vi "RSA FIX.vi"() -> ()   [LabVIEW 2017]
uses:
  <vilib>/Enthought/Python Integration Toolkit/api/Unpack String.vi
  <vilib>/Enthought/Python Integration Toolkit/Python Integration Toolkit.lvlib
panel:
  out "chiptertext":string
  out "plaintext":string
  in  "chipertext":string
  out "Array 2":string[](array[string])
  in  "plaintext":string
  out "error out 3":errorcluster
  out "Array":string[](array[string])
  out "?":string="DESKRIPSI"
  out "error out 2":errorcluster
  out "?":string="DESKRIPSI"
  out "Totient":i64
  in  "e":i64
  out "N":i64
  in  "q":i64
  in  "p":i64
  out "d":i64
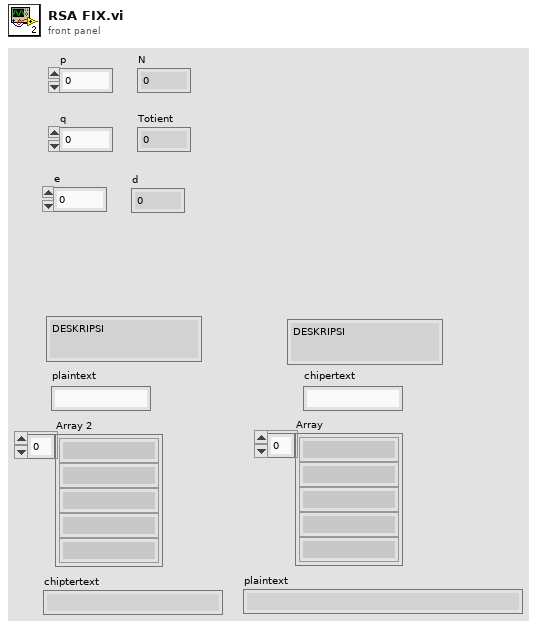
[diagram p1: front panel]
types:
  T1 = typedef "Python Integration Toolkit.lvlib/Session ID.ctl" = u64
  T2 = typedef "Python Integration Toolkit.lvlib/Python Objects.ctl" = variant
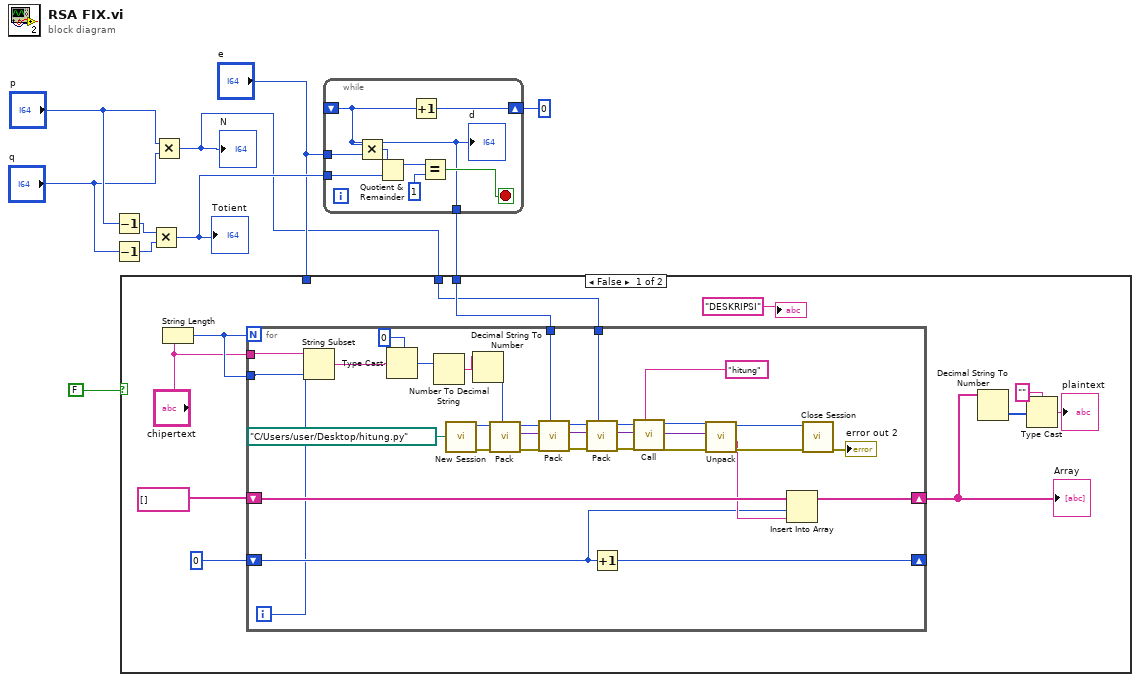
[diagram p0: block diagram]
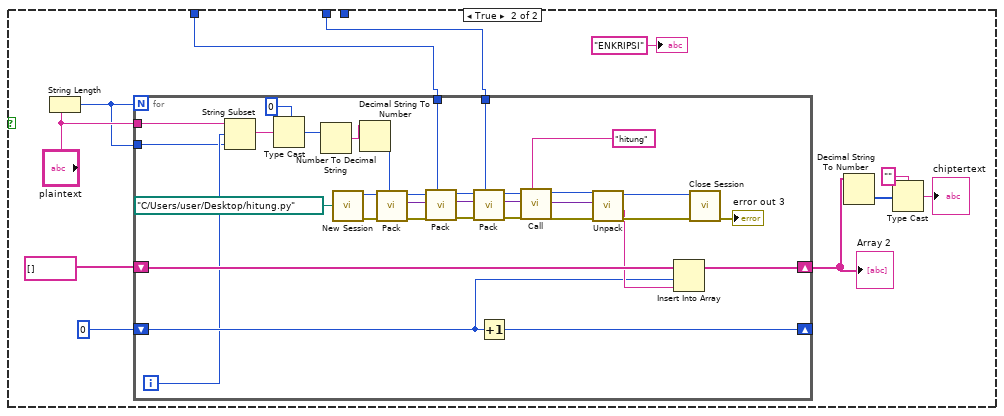
[diagram p2: hidden frame]
diagram:
  n1 = Decrement(x="p") -> (x-1=w6:i64)
  n2 = Decrement(x="q") -> (x-1=w7:i64)
  n3 = Multiply(x=w6, y=w7) -> (x*y=w5:i64)
  "Totient" <- w5
  n4 = Multiply(x="p", y="q") -> (x*y=w3:i64)
  "N" <- w3
  n5 = while {
    shift-right: [w16] -> _
    shift-left: i64 0 -> [w11]
    tunnel: w5 -> [w14]
    tunnel: "e" -> [w13]
    tunnel: [w11] -> w1
    stop <- w18 stop-if-true
    n6 = Multiply(x=w11, y=w13) -> (x*y=w15:i64)
    n7 = Quotient & Remainder(x=w15, y=w14) -> (x-y*floor(x/y)=w17:i64)  [unwired: 1 out]
    n8 = Increment(x=w11) -> (x+1=w16:i64)
    n9 = Equal?(x=w17, y=i64 1) -> (x = y?=w18:bool)
    "d" <- w11
  }
  n10 = case shown="False" FALSE {
    tunnel: "e" -> [_ w68]
    tunnel: w3 -> [w28 w69]
    tunnel: w1 -> [w29 _]
    frame False {
      n11 = String Length(string="chipertext") -> (length=w24:i32)
      n12 = for {
        N: w24 -> [_]
        tunnel: w29 -> [w44]
        tunnel: w28 -> [w43]
        shift-right: [w36] -> w20
        shift-left: string[] [] -> [w38]
        shift-right: [w35] -> _
        shift-left: 0 -> [w34]
        tunnel: "chipertext" -> [w33]
        tunnel: w24 -> [w31]
        i -> [w32]
        n13 = String Subset(string=w33, offset (0)=w32, length (rest)=w31) -> (substring=w30:string)
        n14 = Type Cast(type=u8 0, x=w30) -> (*(type *) &x=w41:u8)
        n15 = Number To Decimal String(number=w41) -> (decimal integer string=w40:string)  [unwired: 1 in]
        n16 = call <vilib>:"New Session.vi"("Path to Python Module (.py File)"=path "C:/Users/user/Desktop/hitung.py") -> ("error out"=w57:errorcluster, "Session ID out"=w62:T1)  [unwired: 9 in]
        n17 = Decimal String To Number(string=w40) -> (number=w39:i32)  [unwired: 2 in, 1 out]
        n18 = call <vilib>:"Pack.vi"("Argument"=w39, "error in (no error)"=w57, "Session ID"=w62) -> ("error out"=w56:errorcluster, "Python Object References Out"=w55:T2, "Session ID out"=w54:T1)  [unwired: 6 in]
        n19 = call <vilib>:"Pack.vi"("Argument"=w44, "error in (no error)"=w56, "Python Object References In"=w55, "Session ID"=w54) -> ("error out"=w48:errorcluster, "Python Object References Out"=w49:T2, "Session ID out"=w50:T1)  [unwired: 5 in]
        n20 = call <vilib>:"Pack.vi"("Argument"=w43, "error in (no error)"=w48, "Python Object References In"=w49, "Session ID"=w50) -> ("error out"=w53:errorcluster, "Python Object References Out"=w52:T2, "Session ID out"=w51:T1)  [unwired: 5 in]
        n21 = Increment(x=w34) -> (x+1=w35:i32)
        n22 = call <vilib>:"Call.vi"("Function or Method Name"="hitung", "error in (no error)"=w53, "Python Object References In"=w52, "Session ID"=w51) -> ("error out"=w46:errorcluster, "Python Object References Out"=w60:T2, "Session ID out"=w61:T1)  [unwired: 5 in]
        n23 = call-poly <vilib>:"Unpack.vi"("error in (no error)"=w46, "Python Object References In"=w60, "Session ID"=w61) -> ("error out"=w58:errorcluster, "Value"=w37:string, "Session ID out"=w59:T1)  [unwired: 5 in, 1 out]
        n24 = Insert Into Array(array=w38, index=w34, new element=w37) -> (w36:string[])
        n25 = call <vilib>:"Close Session.vi"("error in (no error)"=w58, "Session ID"=w59) -> ("error out"=→"error out 2":errorcluster)  [unwired: 9 in]
      }
      "Array" <- w20
      n26 = Decimal String To Number(string=w20) -> (number=w22:i32[])  [unwired: 2 in, 1 out]
      n27 = Type Cast(type="", x=w22) -> (*(type *) &x=→"plaintext":string)
      "?" <- "DESKRIPSI"
    }
    frame True {
      n28 = String Length(string="plaintext") -> (length=w70:i32)
      n29 = for {
        N: w70 -> [_]
        tunnel: w68 -> [w89]
        tunnel: w69 -> [w88]
        shift-right: [w80] -> w65
        shift-left: string[] [] -> [w82]
        shift-right: [w79] -> _
        shift-left: 0 -> [w78]
        tunnel: "plaintext" -> [w76]
        tunnel: w70 -> [w75]
        i -> [w77]
        n30 = String Subset(string=w76, offset (0)=w77, length (rest)=w75) -> (substring=w87:string)
        n31 = Type Cast(type=u8 0, x=w87) -> (*(type *) &x=w85:u8)
        n32 = Number To Decimal String(number=w85) -> (decimal integer string=w84:string)  [unwired: 1 in]
        n33 = call <vilib>:"New Session.vi"("Path to Python Module (.py File)"=path "C:/Users/user/Desktop/hitung.py") -> ("error out"=w102:errorcluster, "Session ID out"=w107:T1)  [unwired: 9 in]
        n34 = Decimal String To Number(string=w84) -> (number=w83:i32)  [unwired: 2 in, 1 out]
        n35 = call <vilib>:"Pack.vi"("Argument"=w83, "error in (no error)"=w102, "Session ID"=w107) -> ("error out"=w101:errorcluster, "Python Object References Out"=w100:T2, "Session ID out"=w99:T1)  [unwired: 6 in]
        n36 = call <vilib>:"Pack.vi"("Argument"=w89, "error in (no error)"=w101, "Python Object References In"=w100, "Session ID"=w99) -> ("error out"=w93:errorcluster, "Python Object References Out"=w94:T2, "Session ID out"=w95:T1)  [unwired: 5 in]
        n37 = call <vilib>:"Pack.vi"("Argument"=w88, "error in (no error)"=w93, "Python Object References In"=w94, "Session ID"=w95) -> ("error out"=w98:errorcluster, "Python Object References Out"=w97:T2, "Session ID out"=w96:T1)  [unwired: 5 in]
        n38 = Increment(x=w78) -> (x+1=w79:i32)
        n39 = call <vilib>:"Call.vi"("Function or Method Name"="hitung", "error in (no error)"=w98, "Python Object References In"=w97, "Session ID"=w96) -> ("error out"=w91:errorcluster, "Python Object References Out"=w105:T2, "Session ID out"=w106:T1)  [unwired: 5 in]
        n40 = call-poly <vilib>:"Unpack.vi"("error in (no error)"=w91, "Python Object References In"=w105, "Session ID"=w106) -> ("error out"=w103:errorcluster, "Value"=w81:string, "Session ID out"=w104:T1)  [unwired: 5 in, 1 out]
        n41 = Insert Into Array(array=w82, index=w78, new element=w81) -> (w80:string[])
        n42 = call <vilib>:"Close Session.vi"("error in (no error)"=w103, "Session ID"=w104) -> ("error out"=→"error out 3":errorcluster)  [unwired: 9 in]
      }
      "Array 2" <- w65
      n43 = Decimal String To Number(string=w65) -> (number=w67:i32[])  [unwired: 2 in, 1 out]
      n44 = Type Cast(type="", x=w67) -> (*(type *) &x=→"chiptertext":string)
      "?" <- "ENKRIPSI"
    }
  }
